vi "Send Stop to Enqueuer Array.vi"(10 "final error code":i32, 11 "Enqueuers":refnum<class "Message Enqueuer.lvclass">[](array[class])) -> ()   [LabVIEW 2016, in "_Parent Actor Template.lvlib" / "_Parent Actor Template.lvclass"]
doc: "Sends a stop command to all the actors referenced in the enqueuer array."
uses:
  _Parent Actor Template.lvclass
  <vilib>/ActorFramework/Message Enqueuer/Message Enqueuer.lvclass
  <vilib>/ActorFramework/Stop Msg/Stop Msg.lvclass/Stop Msg.ctl
  <vilib>/ActorFramework/Message Enqueuer/Message Enqueuer.lvclass/Message Enqueuer.ctl
  <vilib>/ActorFramework/Stop Msg/Send Emergency Stop.vi
  <vilib>/ActorFramework/Stop Msg/Send Normal Stop.vi
  <vilib>/ActorFramework/Message Enqueuer/Enqueue Critical.vi
  <vilib>/ActorFramework/Message Enqueuer/Enqueue.vi
  <vilib>/ActorFramework/Stop Msg/Stop Msg.lvclass
  C:/Program Files (x86)/National Instruments/LabVIEW 2016/vi.lib/ActorFramework/Message/Message.lvclass
  <vilib>/ActorFramework/Message Priority Queue/Priority Enqueue.vi
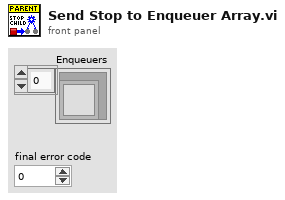
[diagram p1: front panel]
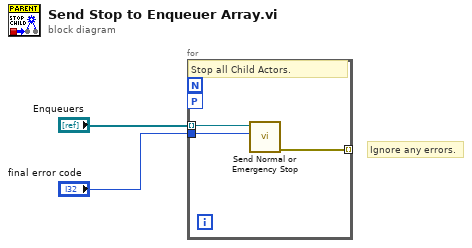
[diagram p0: block diagram]
diagram:
  # "Ignore any errors."
  n1 = for {
    tunnel: "Enqueuers" -> [w5] mode=indexing
    tunnel: [w4] -> _ mode=indexing
    tunnel: "final error code" -> [w3]
    workers-P: _ -> [_]
    # "Stop all Child Actors."
    n2 = call <vilib>:"Send Normal or Emergency Stop.vi"("final error code"=w3, "Message Enqueuer"=w5) -> ("error out"=w4:errorcluster)  [unwired: 9 in]
  }
